vi "Launch Module.vi"(8 "error in":errorcluster) -> (0 "error out":errorcluster)   [LabVIEW 2023, in "Adjust FP VIs.lvlib"]
uses:
  Adjust FP VIs/Adjust FP VIs.lvlib
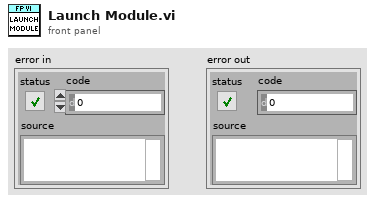
[diagram p1: front panel]
types:
  T1 = enum32{"Invalid", "Standard", "Closed", "Hidden", "Minimized", "Maximized"}
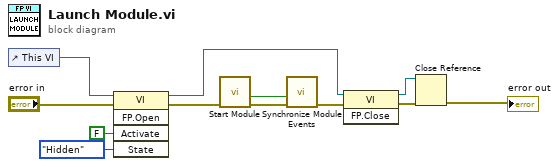
[diagram p0: block diagram]
diagram:
  n1 = control-ref of="This VI"() -> (w10:refnum<vi>)
  n2 = invoke class="VI" method="FP.Open"(reference=w10, error in="error in", "Activate"=FALSE ("Activate?"), "State"=T1."Hidden") -> (reference out=w4:refnum<vi>, error out=w6:errorcluster)  [unwired: 1 in, 3 out]
  n3 = call "Start Module.vi"("error in"=w6) -> ("error out"=w11:errorcluster, "Wait for Event Sync?"=w12:bool)  [unwired: 6 in, 3 out]
  n4 = call "Synchronize Module Events.vi"("error in"=w11, "Wait for Event Sync?"=w12) -> ("error out"=w5:errorcluster)  [unwired: 9 in]
  n5 = invoke class="VI" method="FP.Close"(reference=w4, error in=w5) -> (reference out=w2:refnum<vi>, error out=w3:errorcluster)  [unwired: 1 in, 1 out]
  n6 = Close Reference(reference=w2, error in (no error)=w3) -> (error out=→"error out":errorcluster)
